vi "Default Path.vi"(8 "error in (no error)":errorcluster, 10 "Folder Name [Application Name]":string="Application Name", 11 "Configuration in":refnum<class "Configuration.lvclass">) -> (0 "error out":errorcluster, 3 "Configuration out":refnum<class "Configuration.lvclass">)   [LabVIEW 2019, in "Configuration.lvclass"]
uses:
  Configuration.lvclass
  <vilib>/Utility/sysdir.llb/System Directory Type.ctl
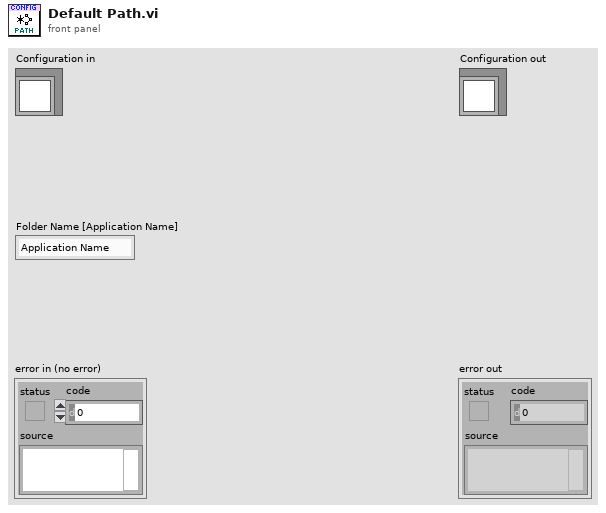
[diagram p1: front panel]
types:
  T1 = typedef "System Directory Type.ctl" = i32
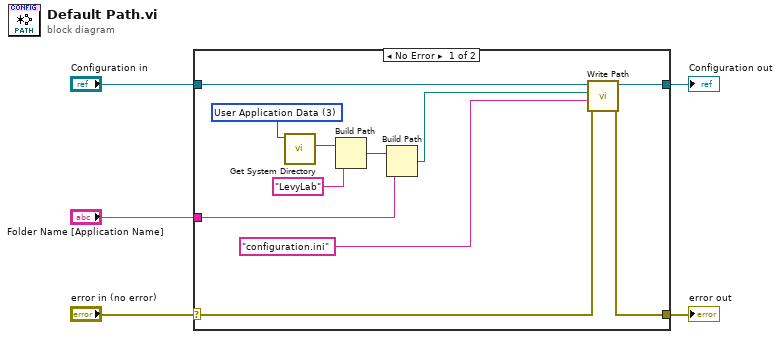
[diagram p0: block diagram]
diagram:
  n1 = case shown="No Error" "error in (no error)" {
    selector: "error in (no error)" -> [w8 w17]
    tunnel: [w7 w17] -> w4
    tunnel: [w9 w18] -> w2
    tunnel: "Configuration in" -> [w10 w18]
    tunnel: "Folder Name [Application Name]" -> [w13 _]
    frame No Error {
      w16 = T1 3 items=["User Home"=0, "User Desktop"=1, "User Documents"=2, "User Application Data"=3, "User Preferences"=4, "User Temporary"=5, "Public Documents"=6, "Public Application Data"=7, "Public Preferences"=8, "Public Cache"=13, "System Core Libraries"=9, "System Installed Libraries"=10, "Application Files"=11, "Boot Volume Root"=12] ("system directory type")
      n2 = call <vilib>:"Get System Directory.vi"("system directory type"=w16) -> ("system directory"=w15:path)  [unwired: 10 in]
      n3 = Build Path(base path=w15, name or relative path="LevyLab") -> (appended path=w14:path)
      n4 = Build Path(base path=w14, name or relative path=w13) -> (appended path=w11:path)
      n5 = call "Write Path.vi"("error in (no error)"=w8, "Filename [Configuration.ini]"="configuration.ini" ("name or relative path"), "Path"=w11, "Configuration in"=w10) -> ("error out"=w7:errorcluster, "Configuration out"=w9:refnum<class "Configuration.lvclass">)  [unwired: 6 in]
    }
    frame Error {
    }
  }
  "error out" <- w4
  "Configuration out" <- w2
